vi "Project Parser Test.vi"(8 "error in (no error)":errorcluster, 11 "file path (use dialog)":path=path "C:/Users/fflores/Documents/GitHub Projects/Project-Documentation-Tool/PDT.lvproj") -> (0 "error out":errorcluster)   [LabVIEW 2020, in "LV Project Items Parser.lvlib"]
uses:
  LV Project Items Parser.lvlib
panel:
  in  "Tree":string(tree)
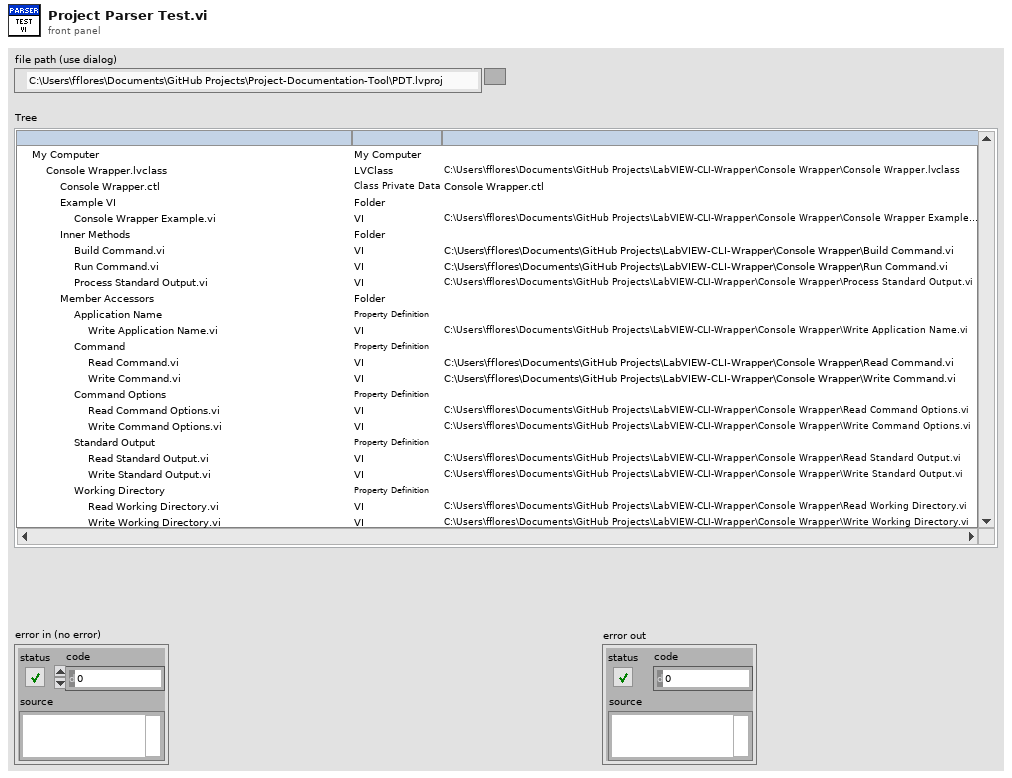
[diagram p1: front panel]
types:
  T1 = cluster{"Left Cell String":string, "Child Text":string[], "Child Tag":string, "Item Indent":i32, "Child Only?":bool, "Glyph Index":i32}[]
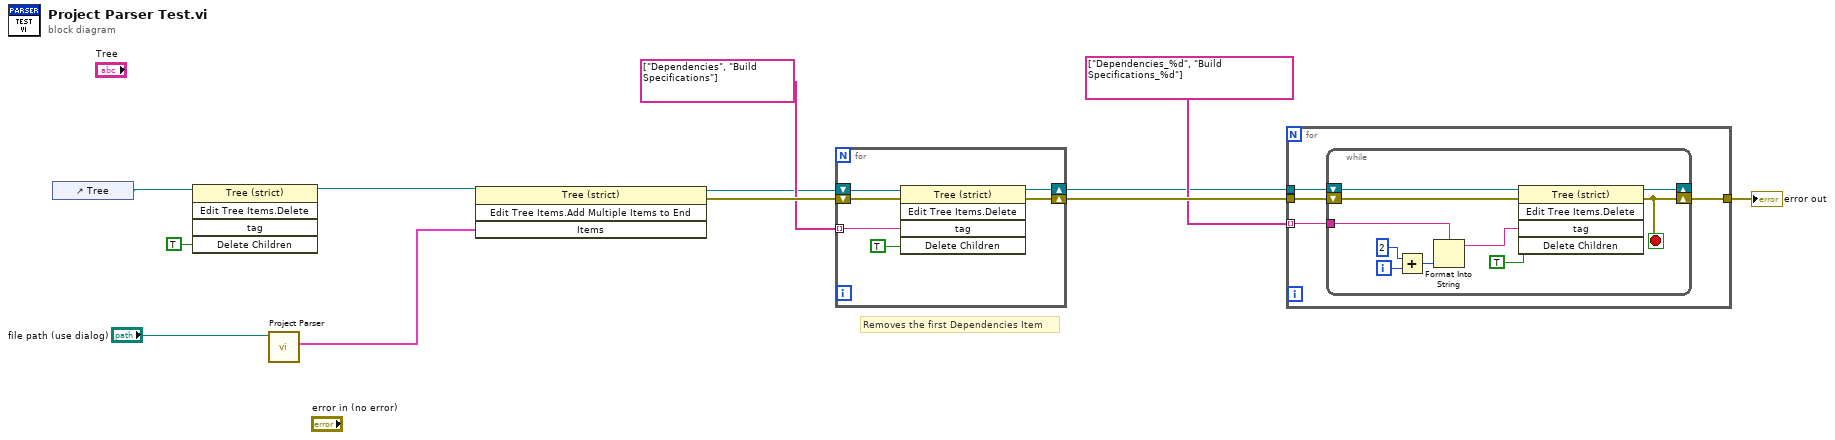
[diagram p0: block diagram]
diagram:
  # "Removes the first Dependencies Item"
  n1 = control-ref of="Tree"() -> (w1:refnum<vi>)
  n2 = invoke on="Invoke Node" class="Tree (strict)" method="Edit Tree Items.Delete"(reference=w1, "Delete Children"=TRUE ("Delete Children?")) -> (reference out=w5:refnum<vi>)  [unwired: 3 in, 4 out]
  n3 = call "Project Parser.vi"("file path (use dialog)"="file path (use dialog)") -> ("Item out"=w6:T1)  [unwired: 9 in, 1 out]
  n4 = invoke on="Invoke Node" class="Tree (strict)" method="Edit Tree Items.Add Multiple Items to End"(reference=w5, "Items"=w6) -> (reference out=w4:refnum<vi>, error out=w11:errorcluster)  [unwired: 2 in, 2 out]
  n5 = for {
    tunnel: string[] ["Dependencies", "Build Specifications"] ("Tag") -> [w16] mode=indexing
    shift-right: [w17] -> w10
    shift-left: w11 -> [w18]
    shift-right: [w13] -> w3
    shift-left: w4 -> [w14]
    n6 = invoke on="Invoke Node" class="Tree (strict)" method="Edit Tree Items.Delete"(reference=w14, error in=w18, "tag"=w16, "Delete Children"=TRUE ("Delete Children?")) -> (reference out=w13:refnum<vi>, error out=w17:errorcluster)  [unwired: 1 in, 3 out]
  }
  n7 = for {
    tunnel: w10 -> [w22]
    tunnel: string[] ["Dependencies_%d", "Build Specifications_%d"] ("Tag") -> [w21] mode=indexing
    tunnel: w3 -> [w20]
    tunnel: [w19] -> w2
    n8 = while {
      tunnel: w21 -> [w26]
      shift-right: [w24] -> _
      shift-left: w20 -> [w25]
      shift-right: [w23] -> w19
      shift-left: w22 -> [w32]
      i -> [w29]
      stop <- w23 stop-if-true
      n9 = Add(x=2, y=w29) -> (x+y=w27:i32)
      n10 = Format Into String(format string=w26, w27) -> (resulting string=w30:string)  [unwired: 2 in, 1 out]
      n11 = invoke on="Invoke Node" class="Tree (strict)" method="Edit Tree Items.Delete"(reference=w25, error in=w32, "tag"=w30, "Delete Children"=TRUE ("Delete Children?")) -> (reference out=w24:refnum<vi>, error out=w23:errorcluster)  [unwired: 1 in, 3 out]
    }
  }
  "error out" <- w2
